vi "Configure Measurement ENR Table.vi"(0 "VISA resource name":refnum<visa-resource-name>, 1 "Enable Common Table (Enabled)":bool=TRUE, 5 "ID for Measurement ENR Table":string, 7 "Serial Number for Measurement ENR Table":string, 9 "Measurement ENR Table Data Entry (Frequency/Amplitude)":dbl[][](array[numeric]), 11 "error in (no error)":errorcluster) -> (4 "VISA resource name out":refnum<visa-resource-name>, 15 "error out":errorcluster)   [LabVIEW 2014, in "Agilent ESA PSA Series.lvlib"]
doc: "Configures the measurement table settings of the Noise Figure personality.\n\n<B>Note:</B> \n\nThis VI is only valid in Noise Figure personality. Use <B>Switch Personality</B> VI to switch to Noise Figure before calling this VI."
uses:
  Agilent ESA PSA Series.lvlib
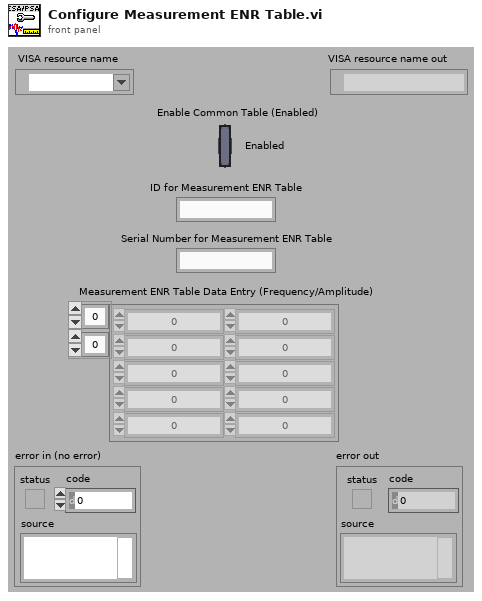
[diagram p1: front panel]
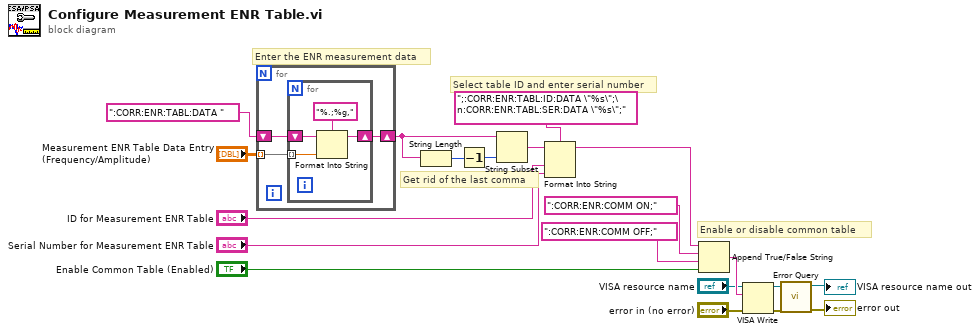
[diagram p0: block diagram]
diagram:
  # "Enable or disable common table"
  # "Get rid of the last comma"
  # "Select table ID and enter serial number"
  # "Enter the ENR measurement data"
  n1 = for {
    tunnel: "Measurement ENR Table Data Entry (Frequency/Amplitude)" -> [w23] mode=indexing
    shift-right: [w21] -> w14
    shift-left: ":CORR:ENR:TABL:DATA " -> [w22]
    n2 = for {
      tunnel: w23 -> [w27] mode=indexing
      shift-right: [w25] -> w21
      shift-left: w22 -> [w26]
      n3 = Format Into String(format string="%.;%g,", initial string=w26, w27) -> (resulting string=w25:string)  [unwired: 1 in, 1 out]
    }
  }
  n4 = String Length(string=w14) -> (length=w15:i32)
  n5 = Decrement(x=w15) -> (x-1=w16:i32)
  n6 = String Subset(string=w14, length (rest)=w16) -> (substring=w3:string)  [unwired: 1 in]
  n7 = Format Into String(format string=";:CORR:ENR:TABL:ID:DATA \"%s\";\n:CORR:ENR:TABL:SER:DATA \"%s\";", initial string=w3, "ID for Measurement ENR Table", "Serial Number for Measurement ENR Table") -> (resulting string=w11:string)  [unwired: 1 in, 1 out]
  n8 = Append True/False String(1:"Enable Common Table (Enabled)", 2:":CORR:ENR:COMM OFF;" ("false string"), 3:":CORR:ENR:COMM ON;" ("true string"), 4:w11) -> (0:w8:string)
  n9 = VISA Write(VISA resource name="VISA resource name", write buffer=w8, error in (no error)="error in (no error)") -> (VISA resource name out=w4:refnum<visa-resource-name>, error out=w6:errorcluster)  [unwired: 1 out]
  n10 = call "Error Query.vi"("error in (no error)"=w6, "VISA resource name"=w4) -> ("error out"=→"error out":errorcluster, "VISA resource name out"=→"VISA resource name out":refnum<visa-resource-name>)  [unwired: 6 in, 2 out]
